vi "Calculate Kinamatics.vi"(2 "y":dbl, 3 "x":dbl) -> (0 "q2":dbl, 1 "q1":dbl)   [LabVIEW 2018]
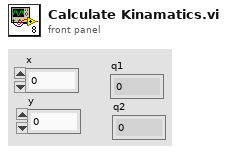
[diagram p1: front panel]
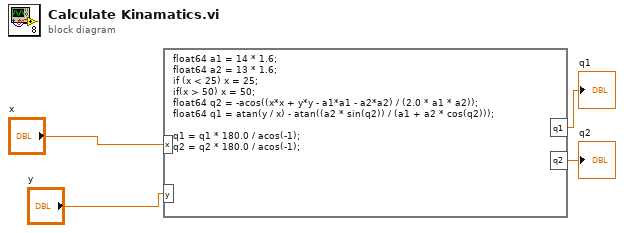
[diagram p0: block diagram]
diagram:
  n1 = formula code="float64 a1 = 14 * 1.6;\nfloat64 a2 = 13 * 1.6;\nif (x < 25) x = 25;\nif(x > 50) x = 50;\nfloat64 q2 = -acos((x*x + y*y - a1*a1 - a2*a2) / (2.0 * a1 * a2));\nfloat64 q1 = atan(y / x) - atan((a2 * sin(q2)) / (a1 + a2 * cos(q2)));\n\nq1 = q1 * 180.0 / acos(-1);\nq2 = q2 * 180.0 / acos(-1);"("x"="x", "y"="y") -> ("q1"=→"q1":dbl, "q2"=→"q2":dbl)
